vi "Live loop.vi"(0 "Camera reference in":refnum<k24>, 5 "Exposure (ms)":dbl=100.0, 7 "Width":i32=2456, 9 "Height":i32=2054, 11 "Error In":errorcluster) -> (4 "Camera reference out":refnum<k24>, 6 "Image Array":u16[][](array[numeric]), 15 "Error Out":errorcluster)   [LabVIEW 2017]
uses:
  C:/Program Files/National Instruments/LabVIEW 2017/instr.lib/IDS/ueye.NET/uEyeDotNet.dll
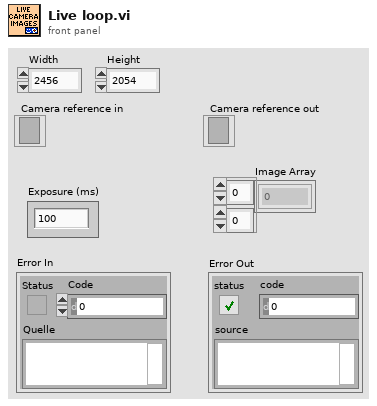
[diagram p1: front panel]
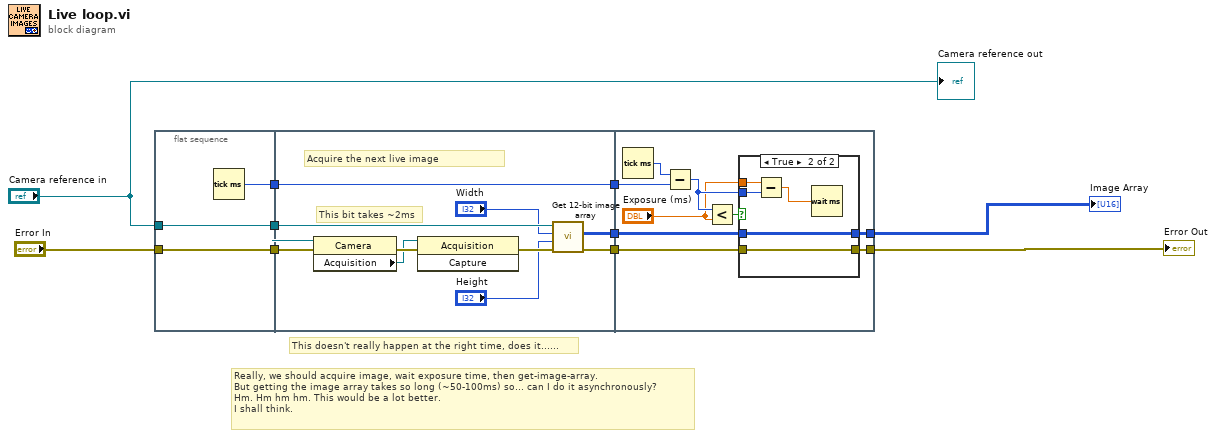
[diagram p0: block diagram]
diagram:
  # "Really, we should acquire image, wait exposure time, then get-image-array.\nBut getting the image array takes so long (~50-100ms) so... can I do it asynchronously? \nHm. Hm hm hm. This would be a lot better. \nI shall think."
  # "This doesn't really happen at the right time, does it......"
  n1 = flat-sequence {
    tunnel: "Error In" -> [w12]
    tunnel: "Camera reference in" -> [w13]
    tunnel: [w13] -> w6
    tunnel: [w12] -> w5
    tunnel: [w11] -> w1
    tunnel: w6 -> [w22]
    tunnel: w5 -> [w21]
    tunnel: [w23] -> w4
    tunnel: [w20] -> w3
    tunnel: [w16] -> w2
    tunnel: w1 -> [w16]
    tunnel: [w27] -> w7
    tunnel: [w29] -> w10
    tunnel: w4 -> [w30]
    tunnel: w3 -> [w28]
    tunnel: w2 -> [w31]
    frame #0 {
      n2 = Tick Count (ms)() -> (millisecond timer value=w11:u32)
    }
    frame #1 {
      # "Acquire the next live image"
      # "This bit takes ~2ms"
      n3 = property class="Camera"(reference=w22, error in=w21) -> (error out=w18:errorcluster, "Acquisition"=w17:refnum<k24>)  [unwired: 1 out]
      n4 = invoke class="Acquisition" method="Capture"(reference=w17, error in=w18) -> (error out=w19:errorcluster)  [unwired: 1 in, 2 out]
      n5 = call "Get 12-bit image array.vi"("Error In"=w19, "Height"="Height", "Width"="Width", "Camera reference in"=w22) -> ("Error Out"=w23:errorcluster, "Array"=w20:u16[][])  [unwired: 4 in, 1 out]
    }
    frame #2 {
      n6 = Tick Count (ms)() -> (millisecond timer value=w32:u32)
      n7 = Subtract(x=w32, y=w31) -> (x-y=w25:u32)
      n8 = Less?(x=w25, y="Exposure (ms)") -> (x < y?=w26:bool)
      n9 = case shown="True" w26 {
        tunnel: [w34 w39] -> w29
        tunnel: w30 -> [w34 w39]
        tunnel: w28 -> [w33 w38]
        tunnel: [w33 w38] -> w27
        tunnel: "Exposure (ms)" -> [_ w36]
        tunnel: w25 -> [_ w35]
        frame False {
        }
        frame True {
          n10 = Subtract(x=w36, y=w35) -> (x-y=w37:dbl)
          n11 = Wait (ms)(milliseconds to wait=w37) -> ()  [unwired: 1 out]
        }
      }
    }
  }
  "Error Out" <- w10
  "Camera reference out" <- "Camera reference in"
  "Image Array" <- w7
